vi "Test_SendAndAskForReply.vi"(8 "error in (no error)":errorcluster) -> (0 "error out":errorcluster)   [LabVIEW 2023]
uses:
  Classes/Communicator/Communicator.lvclass
  <vilib>/addons/_JKI Toolkits/Caraya/classes/Assert/Assert Not Error.vi
  <vilib>/addons/_JKI Toolkits/Caraya/classes/Assert/Assert Equal Value_Variant.vi
  <vilib>/addons/_JKI Toolkits/Caraya/classes/Test/Test.lvclass
  <vilib>/addons/_JKI Toolkits/Caraya/classes/Assert/Assert.lvclass
panel:
  # "Connector Pane"
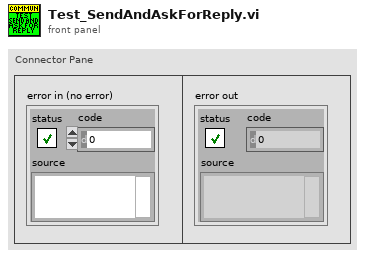
[diagram p1: front panel]
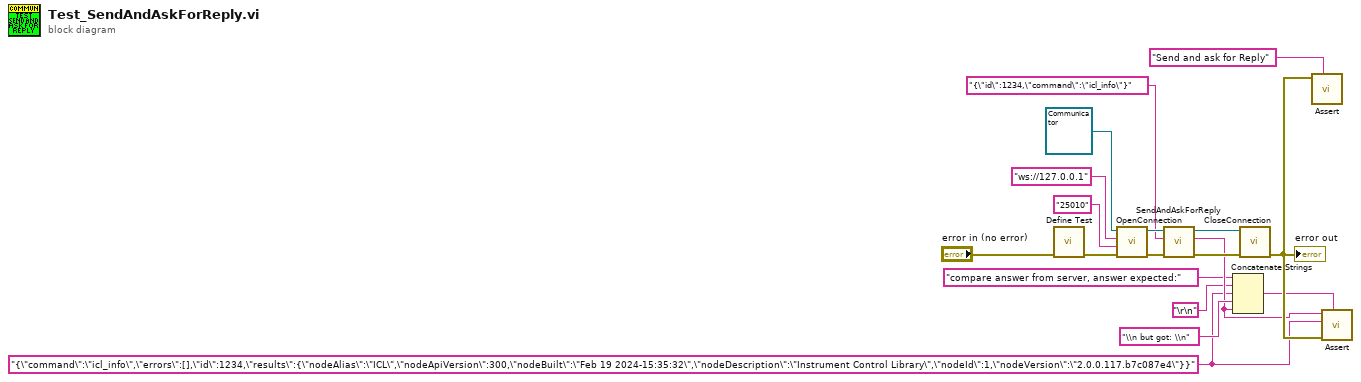
[diagram p0: block diagram]
diagram:
  w1 = "{\"command\":\"icl_info\",\"errors\":[],\"id\":1234,\"results\":{\"nodeAlias\":\"ICL\",\"nodeApiVersion\":300,\"nodeBuilt\":\"Feb 19 2024-15:35:32\",\"nodeDescription\":\"Instrument Control Library\",\"nodeId\":1,\"nodeVersion\":\"2.0.0.117.b7c087e4\"}}" ("test answer from\nwebsocket server")
  n1 = call <vilib>:"Define Test.vi"("error in (no error)"="error in (no error)") -> ("error out"=w15:errorcluster)  [unwired: 9 in, 1 out]
  n2 = call-dynamic "OpenConnection.vi"("error in (no error)"=w15, "WS Server Port"="25010", "WS Server IP"="ws://127.0.0.1", "Communicator in"=refnum<class "Communicator.lvclass"> refnum) -> ("error out"=w12:errorcluster, "Communicator out"=w11:refnum<class "Communicator.lvclass">)  [unwired: 5 in, 1 out]
  n3 = call-dynamic "SendAndAskForReply.vi"("error in (no error)"=w12, "String to be sent"="{\"id\":1234,\"command\":\"icl_info\"}" ("send command"), "Communicator in"=w11) -> ("error out"=w10:errorcluster, "Data"=w5:string, "Communicator out"=w9:refnum<class "Communicator.lvclass">)  [unwired: 6 in]
  n4 = Concatenate Strings("compare answer from server, answer expected:" ("Label"), "\r\n", w1, "\\n but got: \\n" ("string"), w5) -> (w4:string)
  n5 = call-dynamic "CloseConnection.vi"("error in (no error)"=w10, "Communicator in"=w9) -> ("error out"=w8:errorcluster)  [unwired: 8 in, 1 out]
  "error out" <- w8
  n6 = call-poly <vilib>:"Assert.vi"("Label"="Send and ask for Reply", "Not Error?"=w8) -> ()  [unwired: 8 in, 2 out]
  n7 = call-poly <vilib>:"Assert.vi"("Label"=w4, "error in (no error)"=w8, "Y"=w1, "X"=w5) -> ()  [unwired: 6 in, 2 out]
